vi "createTDMSFile.vi"(8 "Error IN":errorcluster caption="constante d'erreur", 10 "TDMS bool":bool, 11 "Répertoire de sortie du fichier TDMS":path) -> (0 "Error OUT":errorcluster caption="constante d'erreur", 1 "Noms voies TDMS":string[](array[string]), 2 "Chemin de sortie TDMS":path, 3 "fichier tdms en sortie":refnum<k34>)   [LabVIEW 2020]
panel:
  out "createFolder?":bool=TRUE
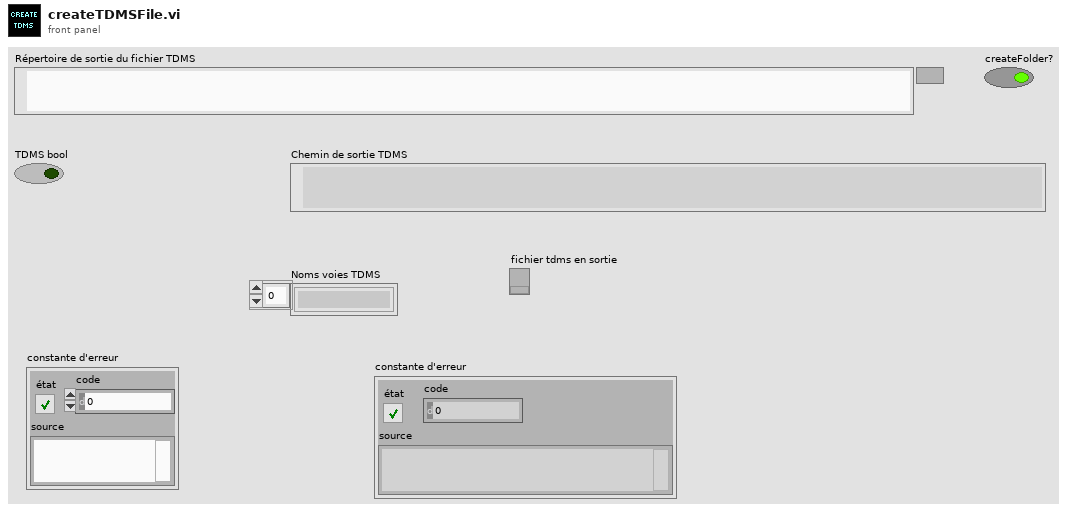
[diagram p1: front panel]
types:
  T1 = enum16{"big-endian, network order", "native, host order", "little-endian"}
  T2 = enum16{"open", "open or create", "create or replace", "create", "open (read-only)"}
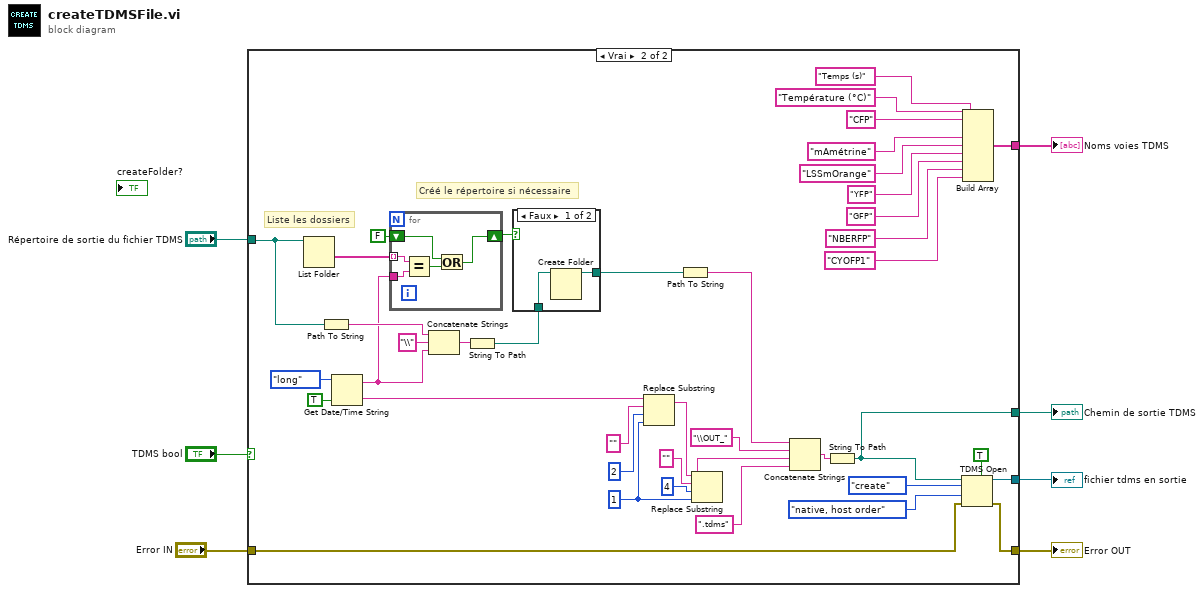
[diagram p0: block diagram]
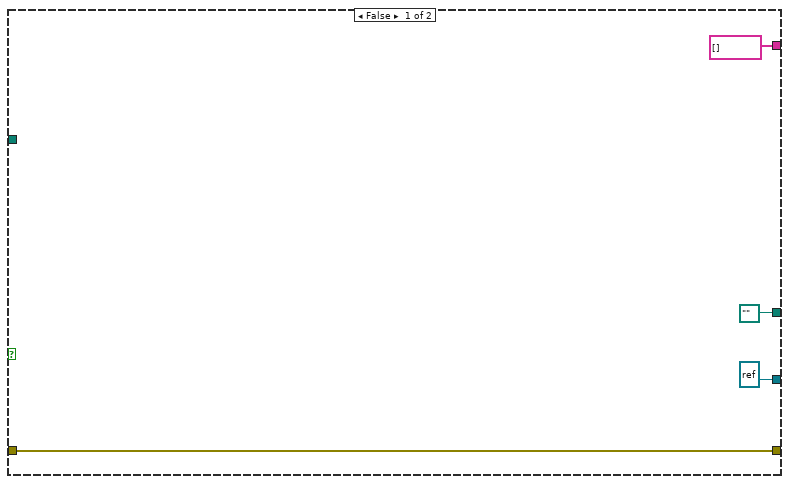
[diagram p2: hidden frame]
diagram:
  n1 = case shown="Vrai" "TDMS bool" {
    tunnel: [string[] [] w32] -> w5
    tunnel: "Répertoire de sortie du fichier TDMS" -> [_ w16]
    tunnel: [refnum<k34> refnum ("tdms file out") w26] -> w4
    tunnel: [path "" w25] -> w3
    tunnel: "Error IN" -> [w8 w24]
    tunnel: [w8 w23] -> w1
    frame False {
    }
    frame True {
      w44 = 1 ("offset (0)")
      # "Créé le répertoire si nécessaire"
      # "Liste les dossiers"
      n2 = List Folder(path=w16) -> (folder names=w21:string[])  [unwired: 3 in, 3 out]
      n3 = Path To String(path=w16) -> (string=w15:string)
      n4 = Get Date/Time String(date format (0)=enum16{"short", "long", "abbreviated"}."long" ("format de date (0)"), want seconds? (F)=TRUE ("secondes ? (F)")) -> (date string=w14:string, time string=w47:string)  [unwired: 1 in]
      n5 = for {
        tunnel: w21 -> [w57] mode=indexing
        tunnel: w14 -> [w56]
        shift-right: [w53] -> w19
        shift-left: FALSE -> [w54]
        n6 = Equal?(x=w57, y=w56) -> (x = y?=w55:bool)
        n7 = Or(x=w54, y=w55) -> (x .or. y?=w53:bool)
      }
      n8 = Concatenate Strings(w15, "\\" ("chaîne"), w14) -> (w13:string)
      n9 = String To Path(string=w13) -> (path=w12:path)
      n10 = case shown="Faux" w19 {
        tunnel: [w59 w60] -> w18
        tunnel: w12 -> [w58 w60]
        frame False {
          n11 = Create Folder(path (use dialog)=w58) -> (created path=w59:path)  [unwired: 2 in, 2 out]
        }
        frame True {
        }
      }
      n12 = Replace Substring(2:w44, 3:2 ("offset (0)"), 4:"" ("sous-chaîne (\"\")"), 5:w47) -> (1:w43:string)  [unwired: 1 out]
      n13 = Path To String(path=w18) -> (string=w22:string)
      n14 = Replace Substring(2:w44, 3:4 ("offset (0)"), 4:"" ("sous-chaîne (\"\")"), 5:w43) -> (1:w31:string)  [unwired: 1 out]
      n15 = Concatenate Strings(w22, "\\OUT_" ("chaîne"), w31, ".tdms" ("chaîne")) -> (w49:string)
      n16 = String To Path(string=w49) -> (path=w25:path)
      n17 = TDMS Open(5:TRUE ("créer un fichier index ? (V)"), 8:w24, 9:T1."native, host order" ("ordre des octets (2 : Little Endian)"), 10:T2."create" ("opération (0 : open)"), 11:w25) -> (0:w23:errorcluster, 3:w26:refnum<k34>)  [unwired: 2 in]
      n18 = Build Array("Temps (s)" ("élément"), "Température (°C)" ("élément"), "CFP" ("élément"), "mAmétrine", "LSSmOrange", "YFP", "GFP" ("élément"), "NBERFP" ("élément"), "CYOFP1" ("élément")) -> (w32:string[])
    }
  }
  "Noms voies TDMS" <- w5
  "fichier tdms en sortie" <- w4
  "Chemin de sortie TDMS" <- w3
  "Error OUT" <- w1
